vi "Get Axis.vi"(8 "error in (no error)":errorcluster, 10 "AcqID":i32, 11 "Automation Refnum in":refnum<k7>) -> (0 "error out":errorcluster, 3 "Spectrum":T1)   [LabVIEW 2014]
uses:
  Spectral Data.ctl
  GetValue Mode.ctl
  PutValue Name.ctl
panel:
  # "LICENSED MATERIALS – PROPERTY OF IBM\nCopyright IBM Corp. 2016,\nALL RIGHTS RESERVED"
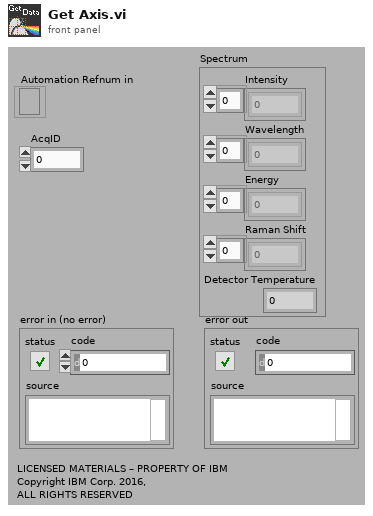
[diagram p1: front panel]
types:
  T1 = typedef "Spectral Data.ctl" = cluster{"Intensity":dbl[], "Wavelength":dbl[], "Energy":dbl[], "Raman Shift":dbl[], "Detector Temperature":dbl}
  T2 = typedef "GetValue Mode.ctl" = enum16{"XY Data", "Data", "MapPoint: Spectrum Index", "Axis Labels", "Axis Units", "Axis", "Axis Index", "Axis Size", "Axis Type", "Intensity", "Frequency", "X", "Y", "Z", "Time", "Double Cursor", "Pointer Limits", "Active Cursors", "Nearest Axis Index", "Acquisition Information", "Custom Information", "History Information", "Data Name", "Dispersion", "Dispersion Parameters", "Labspec Path", "User Level", "System Name", "Autofocus Diode", "Exposure Time", "Live Time", "Labspec Accumulation", "Alignment Diode"}
  T3 = typedef "PutValue Name.ctl" = enum16{"XY Data", "Data", "MapPoint:SpectrumIndex", "Axis Labels", "Axis Units", "Axis", "Axis Limits", "Frequency Unit", "Intensity Unit", "Cursor Type", "Pointer Limits", "Active Cursors", "Special Script Type", "CCD Shutter", "Laser", "SWIFT", "Labspec Exposure Time", "Labspec Accumulation", "Active Frame"}
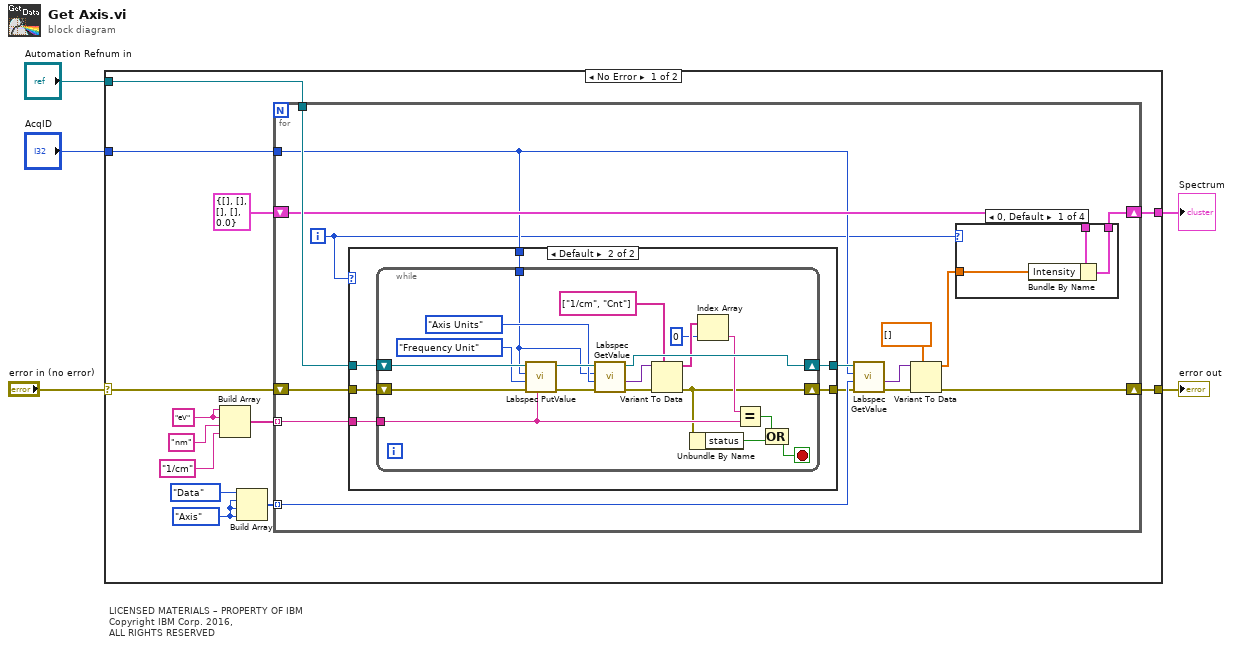
[diagram p0: block diagram]
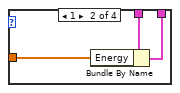
[diagram p2: hidden frame]
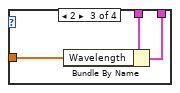
[diagram p3: hidden frame]
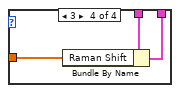
[diagram p4: hidden frame]
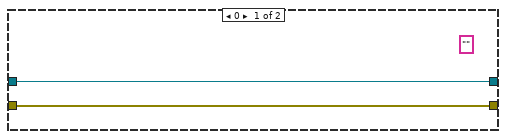
[diagram p5: hidden frame]
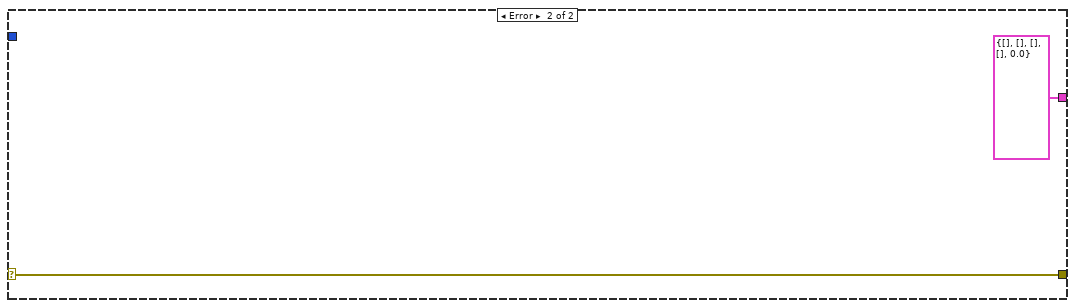
[diagram p6: hidden frame]
diagram:
  # "LICENSED MATERIALS – PROPERTY OF IBM\nCopyright IBM Corp. 2016,\nALL RIGHTS RESERVED"
  n1 = case shown="No Error" "error in (no error)" {
    selector: "error in (no error)" -> [w6 w73]
    tunnel: [w18 w73] -> w5
    tunnel: [w17 T1 {"Intensity"=[], "Wavelength"=[], "Energy"=[], "Raman Shift"=[], "Detector Temperature"=0.0} ("Spectrum")] -> w4
    tunnel: "Automation Refnum in" -> [w8 _]
    tunnel: "AcqID" -> [w7 _]
    frame No Error {
      w14 = GetValue_Mode."Axis" ("Acquisition Mode")
      w9 = "eV"
      n2 = Build Array(w9, w9, "nm", "1/cm") -> (w12:string[])
      n3 = Build Array(GetValue_Mode."Data" ("Acquisition Mode"), w14, w14, w14) -> (w15:T2[])
      n4 = for {
        tunnel: w8 -> [w28]
        tunnel: w12 -> [w31] mode=indexing
        shift-right: [w19] -> w18
        shift-left: w6 -> [w30]
        tunnel: w15 -> [w29] mode=indexing
        shift-right: [w25] -> w17
        shift-left: T1 {"Intensity"=[], "Wavelength"=[], "Energy"=[], "Raman Shift"=[], "Detector Temperature"=0.0} ("Spectrum") -> [w26]
        tunnel: w7 -> [w23]
        i -> [w22]
        n5 = case shown="Default" w22 {
          tunnel: w31 -> [_ w53]
          tunnel: [w47 w48] -> w20
          tunnel: w30 -> [w47 w52]
          tunnel: w28 -> [w46 w51]
          tunnel: [w46 w50] -> w27
          tunnel: w23 -> [_ w49]
          frame 0 {
            (unwired) "" ("Units")
          }
          frame Default {
            n6 = while {
              tunnel: w53 -> [w58]
              tunnel: w49 -> [w66]
              shift-right: [w55] -> w48
              shift-left: w52 -> [w72]
              shift-right: [w69] -> w50
              shift-left: w51 -> [w71]
              stop <- w56 stop-if-true
              n7 = call "Labspec PutValue.vi"("pValue"=w58, "error in"=w72, "Name"=PutValue_Name."Frequency Unit", "DataID"=w66, "Automation Refnum In"=w71) -> ("error out"=w68:errorcluster, "Automation Refnum Out"=w70:refnum<k7>)  [unwired: 1 in, 4 out]
              n8 = call "Labspec GetValue.vi"("error in"=w68, "GetValue Mode"=GetValue_Mode."Axis Units", "DataID"=w66, "Automation Refnum In"=w70) -> ("error out"=w64:errorcluster, "pValue"=w65:variant, "Automation Refnum Out"=w69:refnum<k7>)  [unwired: 1 in, 4 out]
              n9 = Variant To Data(error in=w64, type=string[] ["1/cm", "Cnt"] ("Array 2"), Variant=w65) -> (data=w62:string[], error out=w55:errorcluster)
              n10 = Unbundle By Name(w55) -> ("status"=w54:bool)
              n11 = Index Array(array=w62, index=0) -> (element=w57:string)
              n12 = Equal?(x=w57, y=w58) -> (x = y?=w59:bool)
              n13 = Compound Arithmetic op=OR(w59, w54) -> (w56:bool)
            }
          }
        }
        n14 = call "Labspec GetValue.vi"("error in"=w20, "GetValue Mode"=w29, "DataID"=w23, "Automation Refnum In"=w27) -> ("error out"=w33:errorcluster, "pValue"=w21:variant)  [unwired: 1 in, 5 out]
        n15 = Variant To Data(error in=w33, type=dbl[] [] ("data"), Variant=w21) -> (data=w24:dbl[], error out=w19:errorcluster)
        n16 = case shown="0, Default" w22 {
          tunnel: w26 -> [w36 w39 w42 w45]
          tunnel: [w35 w38 w41 w44] -> w25
          tunnel: w24 -> [w34 w37 w40 w43]
          frame 0, Default {
            n17 = Bundle By Name(cluster=w36, "Intensity"=w34) -> (w35:T1)
          }
          frame 1 {
            n18 = Bundle By Name(cluster=w39, "Energy"=w37) -> (w38:T1)
          }
          frame 2 {
            n19 = Bundle By Name(cluster=w42, "Wavelength"=w40) -> (w41:T1)
          }
          frame 3 {
            n20 = Bundle By Name(cluster=w45, "Raman Shift"=w43) -> (w44:T1)
          }
        }
      }
    }
    frame Error {
    }
  }
  "error out" <- w5
  "Spectrum" <- w4
